vi "FFT Monitor.vi"() -> ()   [LabVIEW 2020]
uses:
  <vilib>/express/express analysis/Spectral/Block/exnSpectralBlock spectral measurements RMS poly.vi
  <vilib>/express/express analysis/Spectral/XNode/ExpressSpectralMeasurementsBlockNode.xnode
  <vilib>/express/express analysis/Spectral/Block/exnSpectralBlock spectral measurements RMS DDT.vi
panel:
  out "task out":refnum<k21>
  in  "timeout (s)":dbl=10.0 format="%0.2f"
  in  "rate":dbl=1600.0
  out "Waveform Graph":dynamicdata(graph)
  out "data":dynamicdata(graph)
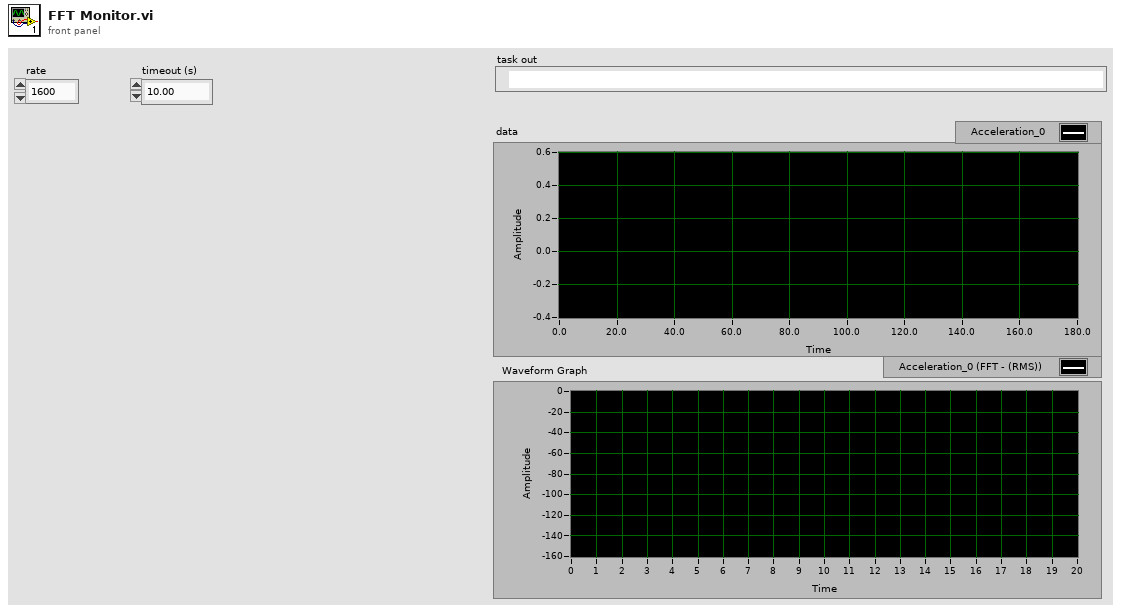
[diagram p1: front panel]
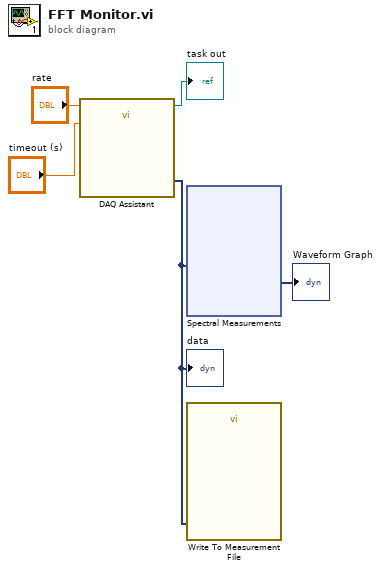
[diagram p0: block diagram]
diagram:
  n1 = call "DAQ Assistant"("rate"="rate", "timeout (s)"="timeout (s)") -> ("task out"=→"task out":refnum<k21>, "data"=w5:dynamicdata, "error out"=w1:errorcluster)  [unwired: 15 in]
  "data" <- w5
  n2 = xnode "Spectral Measurements"("Signals"=w5) -> ("FFT - (RMS)"=→"Waveform Graph":dynamicdata)  [unwired: 1 in, 2 out]
  n3 = call "Write To Measurement File"("Signals"=w5) -> ()  [unwired: 16 in, 3 out]
